vi "accelerometer_test.vi"(7 "Parameters":T2={"Stimulus"={"Type"=enum."Off", "Phase"=0.0, "Amplitude"=[], "Injection point"=enum."Total pose", "Closed loop"=FALSE, "Offset"=[], "Tip -> world"=FALSE, "Frequency"=0.0, "Length"=0.0}, "Goal Filter A"={"Speedup max"=0.0, "Speedup thresh"=0.0, "Speedup nonlin"=0.0, "Filters"=[]}, "Mode controls"={"Hold"=FALSE, "Cancellation"=FALSE, "Goal filter"=FALSE, "Trigger"=FALSE}, "Manipulator type"=enum."Current piezo", "Manipulator calibration"={"Tool offsets"=[[0.0, 0.0, 36200.0]], "Tip light calibration"=[], "Handle light calibration"=[], "Base pivots"=[], "Output pivots"=[], "Length center"=0.0, "Workspace height"=[], "Workspace diameter"=[0.0, 0.0, 36200.0], "Linearization"=[[0.0, 0.0, 36200.0]], "Stack travel"=400.0, "Saturation pos"=375.0, "Inverse filters"=[]}, "Network"={"Remote Host"="", "Send Status"=FALSE, "Send Port"=0, "Recv Commands"=FALSE, "Recv Port"=0}, "Goal Filter B"={"Speedup max"=0.0, "Speedup thresh"=0.0, "Speedup nonlin"=0.0, "Filters"=[]}, "Cancellation"={"KP"={"XY"=0.0, "Rxy"=0.0, "Z"=0.0, "Rz"=0.0}, "KI"=0.0, "KD"={"XY"=0.0, "Rxy"=0.0, "Z"=0.0, "Rz"=0.0}, "Max vel"=20.0, "Max acc"=0.001, "Int error limit"=3.0, "RCM gain"=0.0, "Bypass"=FALSE, "Degraded gain"=0.0}, "Transition time"=0.0, "Estimation"={"Link"={"Measure noise"=[], "Process noise"=[], "Alt process noise"=[], "Alt turnoff cycles"=20, "Innovation limit"=[], "Residue threshold"=0.0, "Enable"=FALSE}, "Handle"={"Measure noise"=[], "Process noise"=[], "State limits"=[], "Innovation limit"=[], "Prediction Lookahead"=0.0, "Enable"=FALSE}}} {"Transition time" format="%_3f"; "Cancellation"."Degraded gain" min=0 max=1 step=0.1 format="%#_3p"; "Cancellation"."RCM gain" min=0 max=1 step=0.1 format="%#_3p"; "Cancellation"."KD"."Rz" min=0 max=1 step=0.1 format="%#_3p"; "Cancellation"."KD"."Rxy" min=0 max=1 step=0.1 format="%#_3p"; "Cancellation"."KD"."Z" min=0 max=1 step=0.1 format="%#_3p"; "Cancellation"."KD"."XY" min=0 max=1 step=0.1 format="%#_3p"; "Cancellation"."KI" min=0 max=1 step=0.01 format="%#_3p"; "Cancellation"."KP"."Rz" min=0 max=1 step=0.1 format="%#_3p"; "Cancellation"."KP"."Rxy" min=0 max=1 step=0.1 format="%#_3p"; "Cancellation"."KP"."Z" min=0 max=1 step=0.1 format="%#_3p"; "Cancellation"."KP"."XY" min=0 max=1 step=0.1 format="%#_3p"; "Cancellation"."Max acc" format="%#_3p"; "Goal Filter B"."Filters"."V limit range" format="%_3p"; "Goal Filter B"."Filters"."V limit" format="%_3p"; "Goal Filter B"."Filters"."Upper Q" format="%_3f"; "Goal Filter B"."Filters"."Upper Fc" format="%_3p"; "Goal Filter B"."Filters"."Lower Q" format="%_3f"; "Goal Filter B"."Filters"."Scale factor" format="%_3f"; "Goal Filter B"."Filters"."Lower Fc" format="%_3p"; "Goal Filter B"."Speedup nonlin" format="%_3p"; "Goal Filter B"."Speedup thresh" format="%_3p"; "Goal Filter B"."Speedup max" format="%_3p"; "Manipulator calibration"."Saturation pos" format="%#.1f"; "Manipulator calibration"."Stack travel" format="%#.1f"; "Manipulator calibration"."Output pivots" format="%#_6f"; "Manipulator calibration"."Base pivots" format="%#_6f"; "Manipulator calibration"."Handle light calibration" format="%#.1f"; "Manipulator calibration"."Tip light calibration" format="%#.1f"; "Goal Filter A"."Filters"."V limit range" format="%_3p"; "Goal Filter A"."Filters"."V limit" format="%_3p"; "Goal Filter A"."Filters"."Upper Q" format="%_3f"; "Goal Filter A"."Filters"."Upper Fc" format="%_3p"; "Goal Filter A"."Filters"."Lower Q" format="%_3f"; "Goal Filter A"."Filters"."Scale factor" format="%_3f"; "Goal Filter A"."Filters"."Lower Fc" format="%_3p"; "Goal Filter A"."Speedup nonlin" format="%_3p"; "Goal Filter A"."Speedup thresh" format="%_3p"; "Goal Filter A"."Speedup max" format="%_3p"; "Stimulus"."Length" min=0.0 max=100.0 step=100.0 format="%#_4p"; "Stimulus"."Frequency" min=0.0 step=100.0 format="%#_4g"; "Stimulus"."Offset" format="%#_3p"; "Stimulus"."Amplitude" format="%#_3p"; "Stimulus"."Phase" min=-180.0 max=360.0 step=100.0 format="%#.2f"}, 10 "Goal Position IN":dbl[][](array[numeric])) -> (2 "Goal Position OUT":dbl[][](array[numeric]))   [LabVIEW 2013]
uses:
  <vilib>/Analysis/Matrix/NI_Matrix.lvlib
  <vilib>/Analysis/Matrix/Numeric/Conversions/Array To Matrix - RA2.vi
  force_control_globals.vi
  <vilib>/Analysis/NI_AALBase.lvlib
  <vilib>/Analysis/baseanly.llb/A x Vector.vi
  testing/injection_point.ctl
  testing/stimulus.ctl
  goal_loop_parms.ctl
  testing/mode_conrols.ctl
  asap/labview/testing/probe_calibration.ctl
  testing/manipulator_cal.ctl
  host/network_params.ctl
  cancellation/decoupled_gain.ctl
  cancellation/sq_control_params.ctl
  cancellation/estimation_controls.ctl
  testing/Micron params.ctl
panel:
  out "Stimulus":dbl[][](array[numeric])=[[0.0, 0.0, 100.0]]
  in  "World Stimulus":dbl[](array[numeric])
  out "Cancellation ON":bool
  out "XY Graph":cluster{"element":dbl, "element":dbl}[](graph)
  in  "Stimulus Type":T1(ring)
  in  "Override with Stimulus":bool
  in  "ASAP Stimulus":dbl[](array[numeric])=[0.0, 0.0, 0.0]
  out "FC Indicator":bool
  in  "Force Control":bool
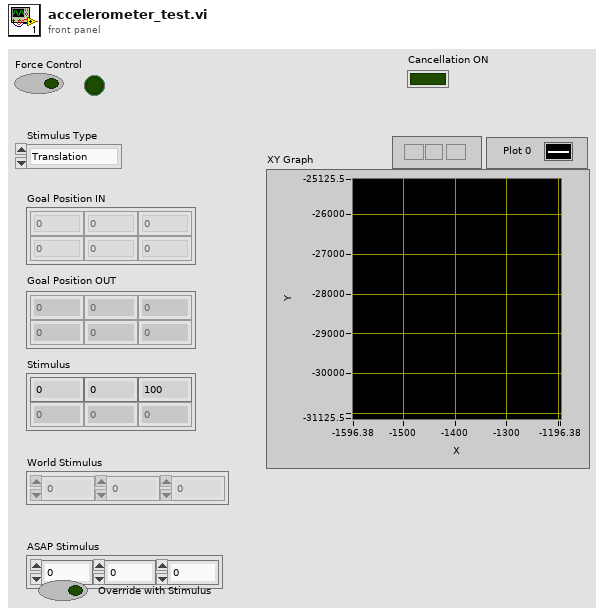
[diagram p1: front panel]
types:
  T1 = enum16{"Translation", "Tip Position", "Rotation"}
  T2 = typedef "Micron params.ctl" = cluster{"Stimulus":T3, "Goal Filter A":T5, "Mode controls":T6, "Manipulator type":enum16{"Current piezo", "Voltage piezo"}, "Manipulator calibration":T7, "Network":T9, "Goal Filter B":T5, "Cancellation":T10, "Transition time":sgl, "Estimation":T12}
  T3 = typedef "stimulus.ctl" = cluster{"Type":enum16{"Off", "Step", "Sine", "Triangle", "Arbitrary"}, "Phase":dbl, "Amplitude":sgl[], "Injection point":T4, "Closed loop":bool, "Offset":sgl[], "Tip -> world":bool, "Frequency":dbl, "Length":dbl}
  T4 = typedef "injection_point.ctl" = enum16{"Total pose", "V limiter", "Goal ", "Link position", "KF link position", "Inverse kin", "Link goal", "Link error", "Controller", "Output", "Drive", "Light"}
  T5 = typedef "goal_loop_parms.ctl" = cluster{"Speedup max":sgl, "Speedup thresh":sgl, "Speedup nonlin":sgl, "Filters":cluster{"Lower Fc":sgl, "Lower Q":sgl, "Scale factor":sgl, "Upper Fc":sgl, "Upper Q":sgl, "V limit":sgl, "V limit range":sgl}[]}
  T6 = typedef "mode_conrols.ctl" = cluster{"Hold":bool, "Cancellation":bool, "Goal filter":bool, "Trigger":bool}
  T7 = typedef "manipulator_cal.ctl" = cluster{"Tool offsets":sgl[][], "Tip light calibration":T8, "Handle light calibration":T8, "Base pivots":sgl[][], "Output pivots":sgl[][], "Length center":sgl, "Workspace height":sgl[], "Workspace diameter":sgl[], "Linearization":sgl[][], "Stack travel":sgl, "Saturation pos":sgl, "Inverse filters":cluster{"filter structure":enum32{"IIR 2nd Order", "IIR 4th Order"}, "Reverse Coefficients":dbl[], "Forward Coefficients":dbl[]}[]}
  T8 = typedef "probe_calibration.ctl" = sgl[][]
  T9 = typedef "network_params.ctl" = cluster{"Remote Host":string, "Send Status":bool, "Send Port":u16, "Recv Commands":bool, "Recv Port":u16}
  T10 = typedef "sq_control_params.ctl" = cluster{"KP":T11, "KI":sgl, "KD":T11, "Max vel":sgl, "Max acc":sgl, "Int error limit":sgl, "RCM gain":sgl, "Bypass":bool, "Degraded gain":sgl}
  T11 = typedef "decoupled_gain.ctl" = cluster{"XY":sgl, "Rxy":sgl, "Z":sgl, "Rz":sgl}
  T12 = typedef "estimation_controls.ctl" = cluster{"Link":cluster{"Measure noise":dbl[], "Process noise":dbl[], "Alt process noise":dbl[], "Alt turnoff cycles":i32, "Innovation limit":dbl[], "Residue threshold":dbl, "Enable":bool}, "Handle":cluster{"Measure noise":dbl[], "Process noise":dbl[], "State limits":dbl[], "Innovation limit":dbl[], "Prediction Lookahead":sgl, "Enable":bool}}
  T13 = typedef "NI_Matrix.lvlib/RealMatrix.ctl" = dbl[][]
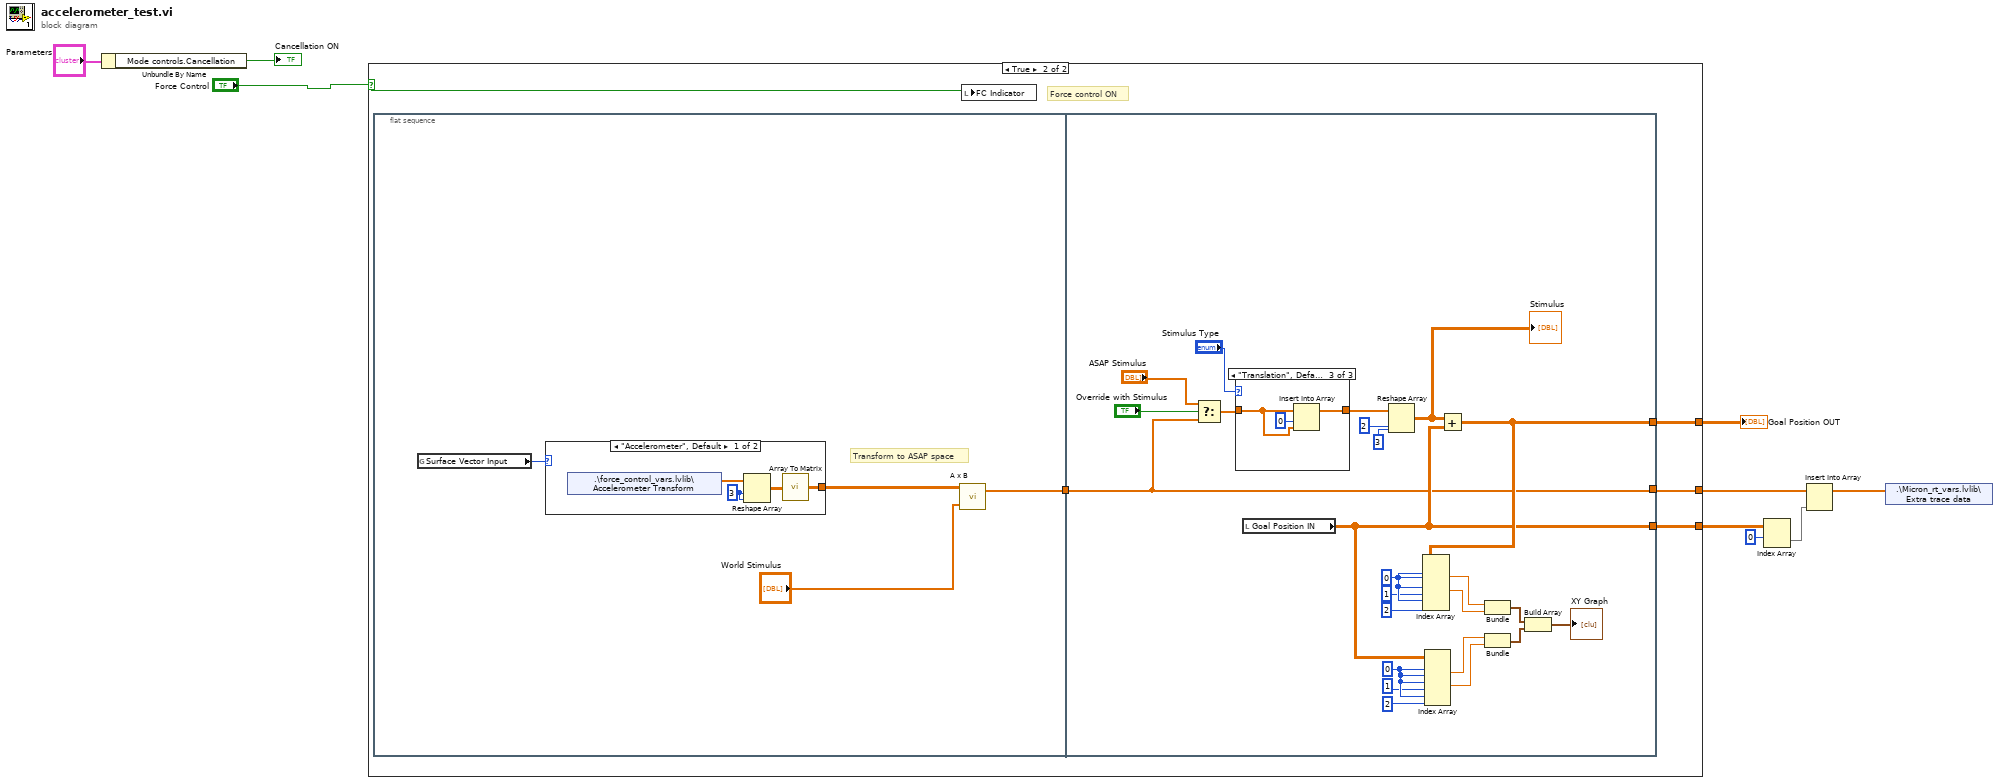
[diagram p0: block diagram]
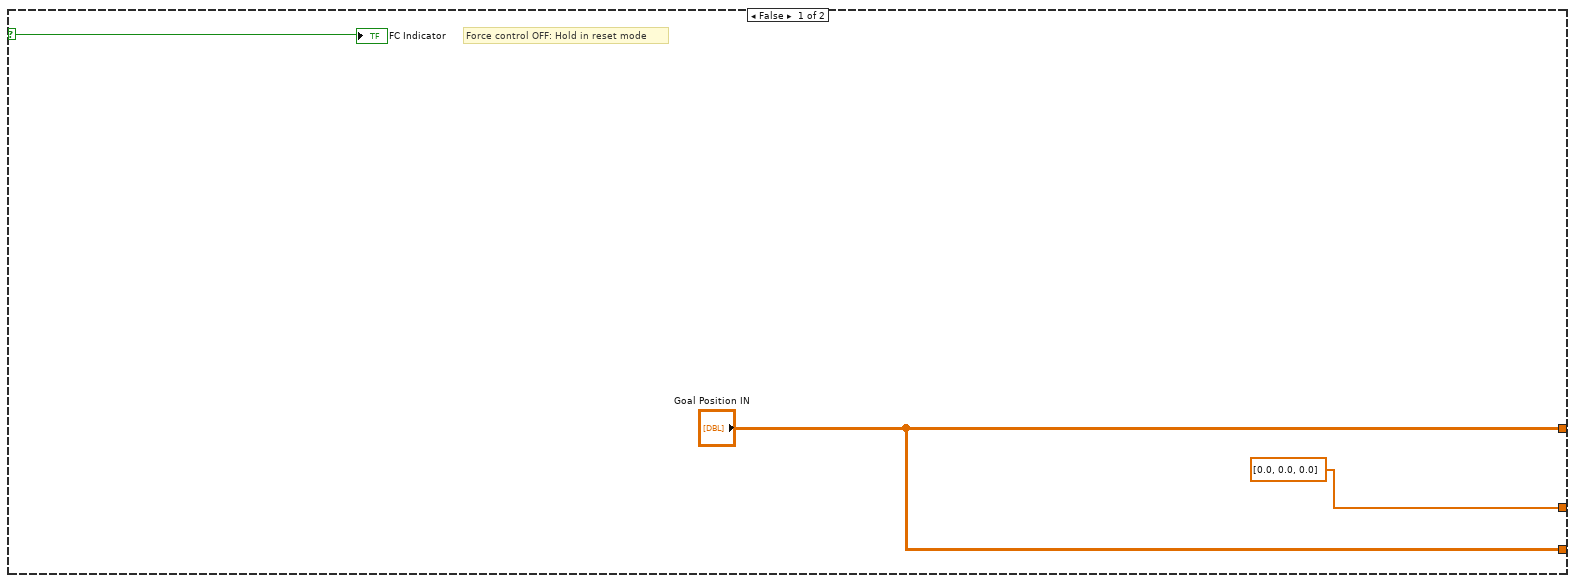
[diagram p2: hidden frame]
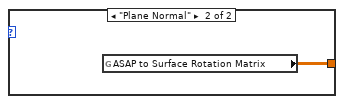
[diagram p3: hidden frame]
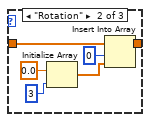
[diagram p5: hidden frame]
diagram:
  n1 = Unbundle By Name("Parameters") -> ("Mode controls.Cancellation"=→"Cancellation ON":bool)
  n2 = case shown="True" "Force Control" {
    selector: "Force Control" -> [w12 w17]
    tunnel: ["Goal Position IN" w16] -> w8
    tunnel: ["Goal Position IN" w14] -> w6
    tunnel: [dbl[] [0.0, 0.0, 0.0] w13] -> w3
    frame False {
      # "Force control OFF: Hold in reset mode"
      "FC Indicator" <- w12
    }
    frame True {
      # "Force control ON"
      n3 = flat-sequence {
        tunnel: [w18] -> w15
        tunnel: [w31] -> w16
        tunnel: [w30] -> w14
        tunnel: [w28] -> w13
        tunnel: w15 -> [w28]
        frame #0 {
          # "Transform to ASAP space"
          n4 = global read "force_control_globals.vi" "Surface Vector Input"() -> (w20:enum16{"Accelerometer", "Plane Normal"})
          n5 = case shown="\"Accelerometer\", Default" w20 {
            tunnel: [w23 w26] -> w21
            frame "Accelerometer", Default {
              w22 = 3 ("dimension size")
              n6 = shared-variable ".\\force_control_vars.lvlib\\Accelerometer Transform"() -> (w25:dbl[])  [unwired: 1 in, 1 out]
              n7 = Reshape Array(w25, w22, w22) -> (w24:dbl[][])
              n8 = call-poly <vilib>:"Array To Matrix.vi"("Real 2D Array"=w24) -> ("Real Matrix"=w23:T13)
            }
            frame "Plane Normal" {
              n9 = global read "force_control_globals.vi" "ASAP to Surface Rotation Matrix"() -> (w26:T13)
            }
          }
          n10 = call-poly <vilib>:"A x B.vi"("Vector"="World Stimulus", "A"=w21) -> ("A x Vector"=w18:dbl[])  [unwired: 1 out]
        }
        frame #1 {
          w37 = 0 ("index")
          w41 = 0 ("index")
          n11 = Select(t="ASAP Stimulus", s="Override with Stimulus", f=w28) -> (s? t:f=w29:dbl[])
          n12 = case shown="\"Translation\", Default" "Stimulus Type" {
            tunnel: [w51 w56 w59] -> w47
            tunnel: w29 -> [w51 w55 w58]
            frame "Tip Position" {
            }
            frame "Rotation" {
              n13 = Initialize Array(0.0 ("element"), 3 ("dimension size")) -> (w54:dbl[])
              n14 = Insert Into Array(array=w55, index=0, new element=w54) -> (w56:dbl[])
            }
            frame "Translation", Default {
              n15 = Insert Into Array(array=w58, index=0, new element=w58) -> (w59:dbl[])
            }
          }
          n16 = local read "Goal Position IN"() -> (w30:dbl[][])
          n17 = Reshape Array(w47, 2, 3) -> (w27:dbl[][])
          "Stimulus" <- w27
          n18 = Index Array(array=w30, index (row) #1=w37, index (col) #1=w37, index (row) #2=w37, index (col) #2=1 ("length"), index (row) #3=w37, index (col) #3=2 ("length")) -> (element #1=w33:dbl, element #2=w32:dbl)  [unwired: 1 out]
          n19 = Add ("Add.vi")(x=w27, y=w30) -> (x+y=w31:dbl[][])
          n20 = Index Array(array=w31, index (row) #1=w41, index (col) #1=w41, index (row) #2=w41, index (col) #2=1 ("length"), index (row) #3=w41, index (col) #3=2 ("length")) -> (element #1=w35:dbl, element #2=w34:dbl)  [unwired: 1 out]
          n21 = Bundle(w35, w34) -> (w43:cluster{dbl, dbl})  [unwired: 1 in]
          n22 = Bundle("Numeric"=w33, "Numeric"=w32) -> (w44:cluster{"Numeric":dbl, "Numeric":dbl})  [unwired: 1 in]
          n23 = Build Array(w43, w44) -> (→"XY Graph":cluster{"Numeric":dbl, "Numeric":dbl}[])
        }
      }
      n24 = local write "FC Indicator"(w17) -> ()
    }
  }
  "Goal Position OUT" <- w8
  n25 = Index Array(array=w6, index (row)=0) -> (element=w5:dbl[])  [unwired: 1 in]
  n26 = Insert Into Array(array=w3, new element=w5) -> (w2:dbl[])  [unwired: 1 in]
  n27 = shared-variable ".\\Micron_rt_vars.lvlib\\Extra trace data"(w2) -> ()  [unwired: 1 in, 1 out]
